vi "Clear.vi"(8 "error in (no error)":errorcluster, 11 "Parameter to Hardware Map in":refnum<class "Parameter to Hardware Map.lvclass">) -> (0 "error out":errorcluster, 3 "Parameter to Hardware Map out":refnum<class "Parameter to Hardware Map.lvclass">)   [LabVIEW 2020, in "RxnRover.lvlib" / "Parameter to Hardware Map.lvclass"]
doc: "Remove all elements from the map, resulting in a size of 0."
uses:
  Parameter to Hardware Map.lvclass
  Parameter to Hardware Map.lvclass/Parameter to Hardware Map.ctl
  Controller/Generic Plugin.lvclass
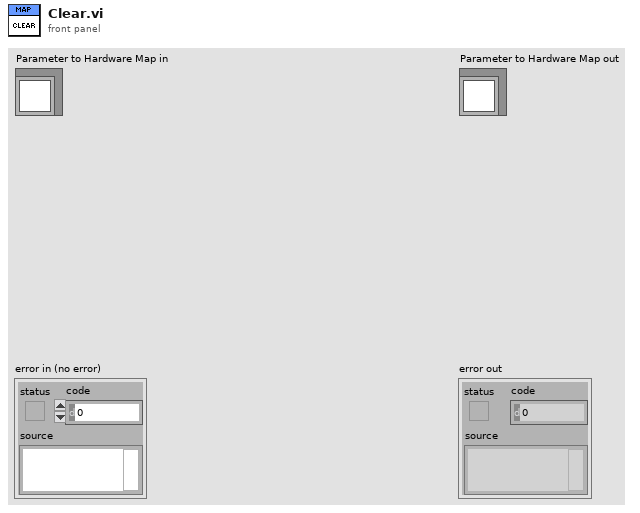
[diagram p1: front panel]
types:
  T1 = typedef "RxnRover.lvlib/Parameter to Hardware Map.lvclass/Pair.ctl" = cluster{"key":string, "values":refnum<class "Generic Plugin.lvclass">[]}
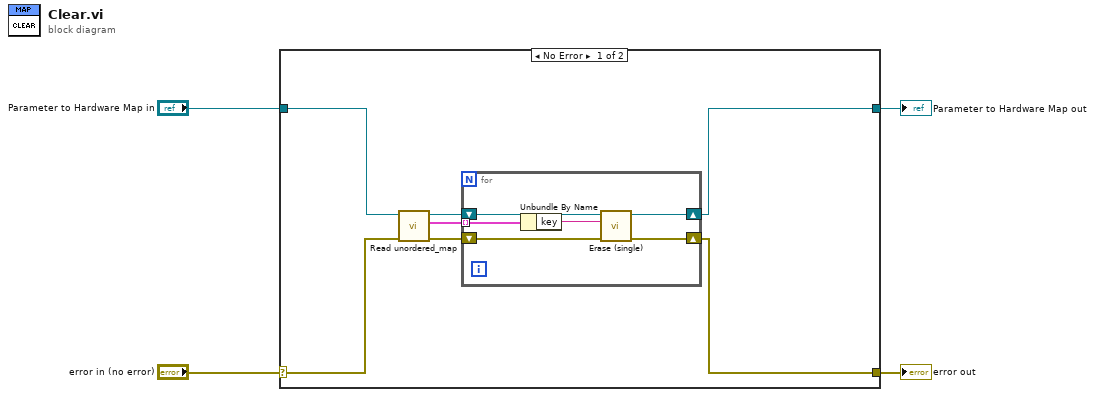
[diagram p0: block diagram]
diagram:
  n1 = case shown="No Error" "error in (no error)" {
    selector: "error in (no error)" -> [w10 w19]
    tunnel: [w6 w19] -> w3
    tunnel: [w5 w18] -> w1
    tunnel: "Parameter to Hardware Map in" -> [w11 w18]
    frame No Error {
      n2 = call "Read unordered_map.vi"("error in (no error)"=w10, "Parameter to Hardware Map in"=w11) -> ("error out"=w7:errorcluster, "unordered_map"=w9:T1[], "Parameter to Hardware Map out"=w8:refnum<class "Parameter to Hardware Map.lvclass">)  [unwired: 7 in]
      n3 = for {
        tunnel: w9 -> [w16] mode=indexing
        shift-right: [w12] -> w5
        shift-left: w8 -> [w17]
        shift-right: [w13] -> w6
        shift-left: w7 -> [w14]
        n4 = Unbundle By Name(w16) -> ("key"=w15:string)
        n5 = call "Erase (single).vi"("error in (no error)"=w14, "Key"=w15, "Parameter to Hardware Map in"=w17) -> ("error out"=w13:errorcluster, "Parameter to Hardware Map out"=w12:refnum<class "Parameter to Hardware Map.lvclass">)  [unwired: 6 in, 1 out]
      }
    }
    frame Error {
    }
  }
  "error out" <- w3
  "Parameter to Hardware Map out" <- w1
